vi "Autonomous Independent.vi"   [LabVIEW 2015]
doc: "This VI is called when autonomous begins, and will automatically be terminated when autonomous ends. You can carry out timed or sensor driven robot movement independently without needing to return to the caller."
uses:
  <vilib>/Rock Robotics/WPI/Utilities/WPI_GetSetVariantRefNum.vi
  <vilib>/Rock Robotics/Network Tables/SD Write Numeric Array.vi
  <vilib>/Rock Robotics/Network Tables/SD Read Number.vi
  <vilib>/Rock Robotics/WPI/RobotDrive/WPI_RobotDriveMecanumDrive_Cartesian.vi
panel:
  # "Be sure to right-click and choose Data Operations>>Make Current Value default if you want to save the array values with the VI"
types:
  T1 = typedef "WPI_JoystickDevRef.ctl" = cluster{"Device":T2}
  T2 = typedef "WPI_JoystickDeviceEnum.ctl" = enum16{"USB 0", "USB 1", "USB 2", "USB 3", "USB 4", "USB 5"}
  T3 = typedef "WPI_GyroDevRef.ctl" = cluster{"DevStatus":errorcluster, "Analog Channel":T4, "Offset":dbl, "Gain (VoltsPerDegree/Second)":dbl, "Gyro Type":enum16{"Analog", "XRS450"}, "Handle":i32, "SPI Bus":T5, "Device Found":bool, "Sample Rate":dbl, "Calibrate On Open":bool}
  T4 = typedef "FPGA_AIChannel.ctl" = enum8{"AI 0", "AI 1", "AI 2", "AI 3", "AI MXP 0", "AI MXP 1", "AI MXP 2", "AI MXP 3", "Invalid"}
  T5 = typedef "spi_bus.ctl" = enum16{"SPI On-Board, CS0", "SPI On-Board, CS1", "SPI On-Board, CS2", "SPI On-Board, CS3", "SPI MXP", "Invalid"}
  T6 = typedef "WPI_MotorControlDeviceRef.ctl" = cluster{"DeviceStatus":errorcluster, "Type":T7, "PWM":cluster{"PWM Channel":T8, "DeadBand":T9}, "CAN":cluster{"Device Number":u8, "Control Mode":T10, "Semaphore":T11, "Max Vout":dbl, "TalonSRX Control Mode":T12}, "Invert":bool}
  T7 = typedef "WPI_MotorControlType.ctl" = enum16{"PWM", "CAN", "CANTalonSRX"}
  T8 = typedef "FPGA_DIOPWMChannel.ctl" = enum8{"PWM 0", "PWM 1", "PWM 2", "PWM 3", "PWM 4", "PWM 5", "PWM 6", "PWM 7", "PWM 8", "PWM 9", "PWM MXP 0", "PWM MXP 1", "PWM MXP 2", "PWM MXP 3", "PWM MXP 4", "PWM MXP 5", "PWM MXP 6", "PWM MXP 7", "PWM MXP 8", "PWM MXP 9", "Invalid"}
  T9 = typedef "WPI_PWMDeadband.ctl" = cluster{"Name":string, "maxPositivePwm":i32, "minPositivePwm":i32, "centerPwm":i32, "maxNegativePwm":i32, "minNegativePwm":i32, "angularRange":u16}
  T10 = typedef "WPI_CANJaguar_ControlMode.ctl" = enum8{"Percent VBus", "Current", "Speed", "Position", "Voltage"}
  T11 = typedef "Semaphore RefNum" = refnum<k1>
  T12 = typedef "WPI_CANTalonSRX_APIControlMode.ctl" = enum8{"Percent VBus", "Speed", "Position", "Slave", "Unchanged / Invalid", "Voltage Compensation", "Current", "Motion Profile"}
  T13 = typedef "WPI_RobotDriveDevRef.ctl" = cluster{"DevStatus":errorcluster, "Motors[]":T6[], "Square Inputs":bool, "Max Output":dbl}
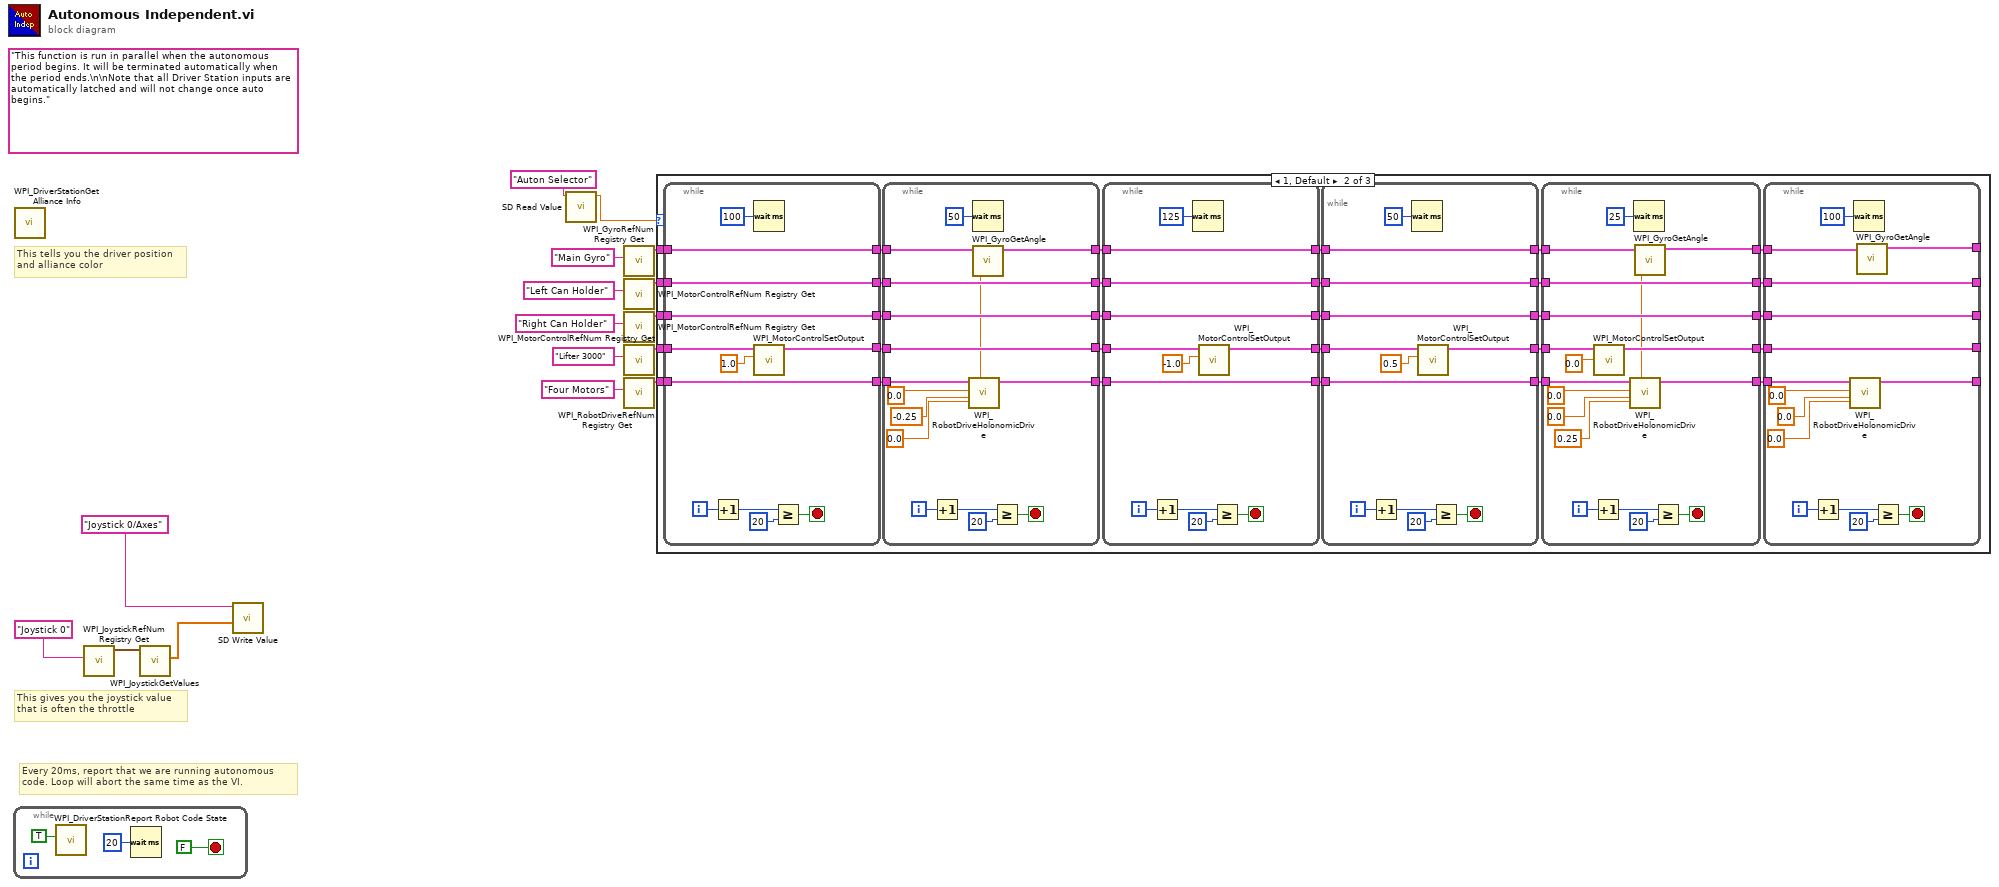
[diagram p0: block diagram]
diagram:
  (unwired) "This function is run in parallel when the autonomous period begins. It will be terminated automatically when the period ends.\n\nNote that all Driver Station inputs are automatically latched and will not change once auto begins."
  # "Every 20ms, report that we are running autonomous\ncode. Loop will abort the same time as the VI."
  # "This gives you the joystick value\nthat is often the throttle"
  # "This tells you the driver position\nand alliance color"
  n1 = while {
    stop <- FALSE stop-if-true
    n2 = call <vilib>:"WPI_DriverStationReport Robot Code State.vi"("Autonomous"=TRUE) -> ()  [unwired: 10 in, 1 out]
    n3 = Wait (ms)(milliseconds to wait=u32 20) -> ()  [unwired: 1 out]
  }
  n4 = call <vilib>:"WPI_DriverStationGet Alliance Info.vi"() -> ()  [unwired: 12 out]
  n5 = call <vilib>:"WPI_JoystickRefNum Registry Get.vi"("refnum name"="Joystick 0") -> ("JoystickDevRef"=w15:T1)  [unwired: 1 in, 9 out]
  n6 = call <vilib>:"WPI_JoystickGetValues.vi"("JoystickDevRef"=w15) -> ("Axes"=w13:dbl[])  [unwired: 6 in, 4 out]
  n7 = call-poly <vilib>:"SD Write Value.vi"("Numeric Array"=w13, "Name"="Joystick 0/Axes") -> ()  [unwired: 8 in, 2 out]
  n8 = call-poly <vilib>:"SD Read Value.vi"("Name"="Auton Selector") -> ("Numeric"=w12:dbl)  [unwired: 8 in, 2 out]
  n9 = call <vilib>:"WPI_GyroRefNum Registry Get.vi"("refnum name"="Main Gyro") -> ("GyroDevRef"=w2:T3)  [unwired: 9 in, 1 out]
  n10 = call <vilib>:"WPI_MotorControlRefNum Registry Get.vi"("refnum name"="Left Can Holder") -> ("MotorControlDevRef"=w10:T6)  [unwired: 9 in, 1 out]
  n11 = call <vilib>:"WPI_MotorControlRefNum Registry Get.vi"("refnum name"="Right Can Holder") -> ("MotorControlDevRef"=w9:T6)  [unwired: 9 in, 1 out]
  n12 = call <vilib>:"WPI_MotorControlRefNum Registry Get.vi"("refnum name"="Lifter 3000") -> ("MotorControlDevRef"=w8:T6)  [unwired: 9 in, 1 out]
  n13 = call <vilib>:"WPI_RobotDriveRefNum Registry Get.vi"("refnum name"="Four Motors") -> ("RobotDriveDevRef"=w7:T13)  [unwired: 9 in, 1 out]
  n14 = case shown="1, Default" w12 {
    tunnel: w10 -> [_ w49 _]
    tunnel: w9 -> [_ w48 _]
    tunnel: w8 -> [_ w47 _]
    tunnel: w7 -> [_ w46 _]
    tunnel: w2 -> [_ w45 _]
    frame 0 {
    }
    frame 1, Default {
      n15 = while {
        tunnel: w49 -> [w129]
        tunnel: w48 -> [w130]
        tunnel: w47 -> [w126]
        tunnel: w46 -> [w127]
        tunnel: [w130] -> w42
        tunnel: [w129] -> w43
        tunnel: w45 -> [w123]
        tunnel: [w123] -> w44
        tunnel: [w127] -> w40
        tunnel: [w125] -> w41
        i -> [w134]
        stop <- w131 stop-if-true
        n16 = Increment(x=w134) -> (x+1=w133:i32)
        n17 = Wait (ms)(milliseconds to wait=u32 100) -> ()  [unwired: 1 out]
        n18 = call <vilib>:"WPI_MotorControlSetOutput.vi"("Output"=1.0, "MotorControlDevRef"=w126) -> ("MotorControlDevRef"=w125:T6)  [unwired: 7 in, 2 out]
        n19 = Greater Or Equal?(x=w133, y=20) -> (x >= y?=w131:bool)
      }
      n20 = while {
        tunnel: w43 -> [w117]
        tunnel: w42 -> [w118]
        tunnel: w41 -> [w115]
        tunnel: w40 -> [w114]
        tunnel: [w118] -> w37
        tunnel: [w117] -> w36
        tunnel: w44 -> [w109]
        tunnel: [w108] -> w35
        tunnel: [w115] -> w38
        tunnel: [w113] -> w39
        i -> [w122]
        stop <- w119 stop-if-true
        n21 = Increment(x=w122) -> (x+1=w121:i32)
        n22 = Wait (ms)(milliseconds to wait=u32 50) -> ()  [unwired: 1 out]
        n23 = call <vilib>:"WPI_GyroGetAngle.vi"("GyroDevRef"=w109) -> ("Angle"=w107:dbl, "GyroDevRef"=w108:T3)  [unwired: 6 in, 3 out]
        n24 = call-poly <vilib>:"WPI_RobotDriveHolonomicDrive.vi"("Rotation"=0.0 ("X"), "Gyro Angle"=w107, "Y"=-0.25 ("X"), "X"=0.0, "RobotDriveDevRef"=w114) -> ("RobotDriveDevRef"=w113:T13)  [unwired: 4 in, 2 out]
        n25 = Greater Or Equal?(x=w121, y=20) -> (x >= y?=w119:bool)
      }
      n26 = while {
        tunnel: w36 -> [w101]
        tunnel: w37 -> [w102]
        tunnel: w38 -> [w96]
        tunnel: w39 -> [w98]
        tunnel: [w102] -> w32
        tunnel: [w101] -> w31
        tunnel: w35 -> [w99]
        tunnel: [w99] -> w30
        tunnel: [w98] -> w34
        tunnel: [w95] -> w33
        i -> [w106]
        stop <- w103 stop-if-true
        n27 = Increment(x=w106) -> (x+1=w105:i32)
        n28 = Wait (ms)(milliseconds to wait=u32 125) -> ()  [unwired: 1 out]
        n29 = call <vilib>:"WPI_MotorControlSetOutput.vi"("Output"=-1.0, "MotorControlDevRef"=w96) -> ("MotorControlDevRef"=w95:T6)  [unwired: 7 in, 2 out]
        n30 = Greater Or Equal?(x=w105, y=20) -> (x >= y?=w103:bool)
      }
      n31 = while {
        tunnel: w31 -> [w89]
        tunnel: w32 -> [w90]
        tunnel: w33 -> [w84]
        tunnel: w34 -> [w86]
        tunnel: [w90] -> w27
        tunnel: [w89] -> w26
        tunnel: w30 -> [w87]
        tunnel: [w87] -> w25
        tunnel: [w86] -> w29
        tunnel: [w83] -> w28
        i -> [w94]
        stop <- w91 stop-if-true
        n32 = Increment(x=w94) -> (x+1=w93:i32)
        n33 = Wait (ms)(milliseconds to wait=u32 50) -> ()  [unwired: 1 out]
        n34 = call <vilib>:"WPI_MotorControlSetOutput.vi"("Output"=0.5, "MotorControlDevRef"=w84) -> ("MotorControlDevRef"=w83:T6)  [unwired: 7 in, 2 out]
        n35 = Greater Or Equal?(x=w93, y=20) -> (x >= y?=w91:bool)
      }
      n36 = while {
        tunnel: w26 -> [w77]
        tunnel: w27 -> [w78]
        tunnel: w28 -> [w70]
        tunnel: w29 -> [w75]
        tunnel: [w78] -> w22
        tunnel: [w77] -> w21
        tunnel: w25 -> [w67]
        tunnel: [w66] -> w20
        tunnel: [w69] -> w23
        tunnel: [w74] -> w24
        i -> [w82]
        stop <- w79 stop-if-true
        n37 = Increment(x=w82) -> (x+1=w81:i32)
        n38 = call <vilib>:"WPI_MotorControlSetOutput.vi"("Output"=0.0, "MotorControlDevRef"=w70) -> ("MotorControlDevRef"=w69:T6)  [unwired: 7 in, 2 out]
        n39 = Wait (ms)(milliseconds to wait=u32 25) -> ()  [unwired: 1 out]
        n40 = call <vilib>:"WPI_GyroGetAngle.vi"("GyroDevRef"=w67) -> ("Angle"=w65:dbl, "GyroDevRef"=w66:T3)  [unwired: 6 in, 3 out]
        n41 = call-poly <vilib>:"WPI_RobotDriveHolonomicDrive.vi"("Rotation"=0.25 ("X"), "Gyro Angle"=w65, "Y"=0.0 ("X"), "X"=0.0, "RobotDriveDevRef"=w75) -> ("RobotDriveDevRef"=w74:T13)  [unwired: 4 in, 2 out]
        n42 = Greater Or Equal?(x=w81, y=20) -> (x >= y?=w79:bool)
      }
      n43 = while {
        tunnel: w21 -> [w59]
        tunnel: w22 -> [w60]
        tunnel: w23 -> [w57]
        tunnel: w24 -> [w56]
        tunnel: [w60] -> _
        tunnel: [w59] -> _
        tunnel: w20 -> [w51]
        tunnel: [w57] -> _
        tunnel: [w55] -> _
        tunnel: [w50] -> _
        i -> [w64]
        stop <- w61 stop-if-true
        n44 = Increment(x=w64) -> (x+1=w63:i32)
        n45 = call-poly <vilib>:"WPI_RobotDriveHolonomicDrive.vi"("Rotation"=0.0 ("X"), "Y"=0.0 ("X"), "X"=0.0, "RobotDriveDevRef"=w56) -> ("RobotDriveDevRef"=w55:T13)  [unwired: 5 in, 2 out]
        n46 = Wait (ms)(milliseconds to wait=u32 100) -> ()  [unwired: 1 out]
        n47 = call <vilib>:"WPI_GyroGetAngle.vi"("GyroDevRef"=w51) -> ("GyroDevRef"=w50:T3)  [unwired: 6 in, 4 out]
        n48 = Greater Or Equal?(x=w63, y=20) -> (x >= y?=w61:bool)
      }
    }
    frame 2 {
    }
  }
